vi "Create Default Attributes.vi"(5 "Unique ID":string, 7 "Process Executive Ref":refnum<data-value>, 11 "iProcess Step Model in":refnum<class "iProcess Step Model.lvclass">) -> (3 "iProcess Step Model out":refnum<class "iProcess Step Model.lvclass">)   [LabVIEW 2019, in "iProcess Step Model.lvclass"]
uses:
  <vilib>/gpm_packages/@cs/Car-wash/Source/iProcess Step Model/iProcess Step Model/iProcess Step Model.lvclass
  <vilib>/gpm_packages/@cs/test-executive/Source/Test Executive/ITestExecutive/ITest Executive.lvclass
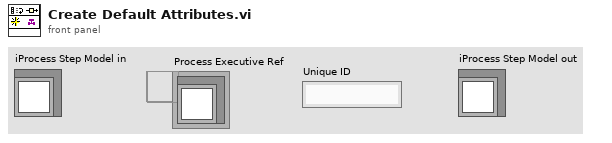
[diagram p1: front panel]
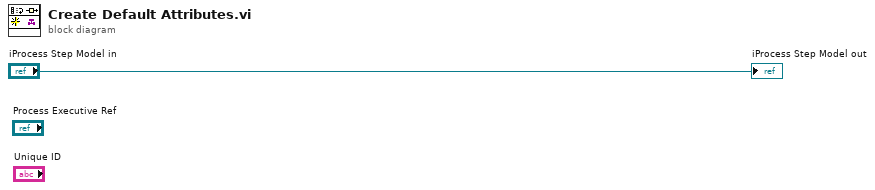
[diagram p0: block diagram]
diagram:
  "iProcess Step Model out" <- "iProcess Step Model in"
